vi "GDSLvIcon_GenerateShortClassIconName.vi"(10 "Rows(1)":u8=1, 11 "ClassName":string) -> (3 "ShortClassIconName":string)   [LabVIEW 2012]
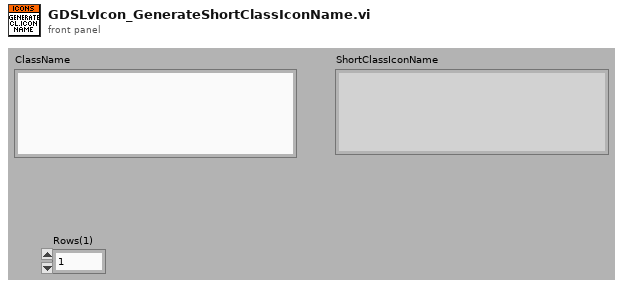
[diagram p1: front panel]
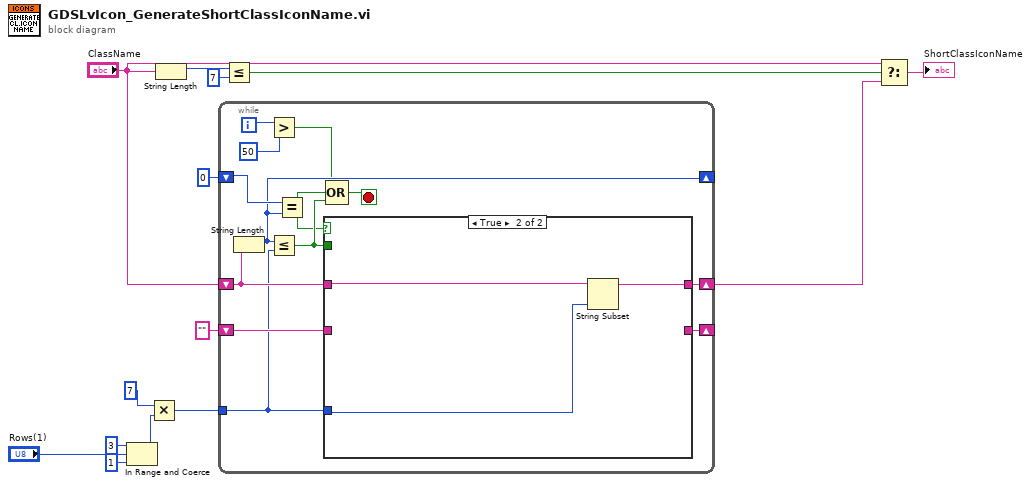
[diagram p0: block diagram]
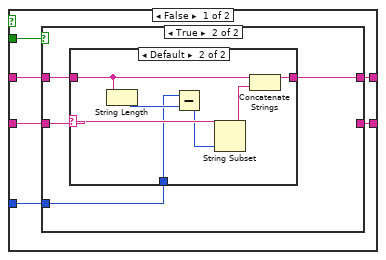
[diagram p2: hidden frame]
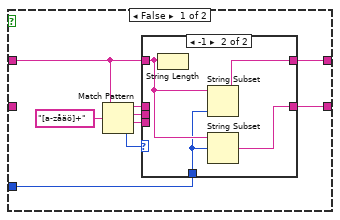
[diagram p3: hidden frame]
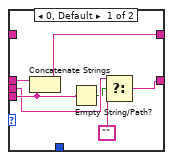
[diagram p4: hidden frame]
diagram:
  n1 = In Range and Coerce(upper limit=u8 3, x="Rows(1)", lower limit=u8 1) -> (coerced(x)=w3:u8)  [unwired: 1 out]
  n2 = Multiply(x=7 ("y"), y=w3) -> (x*y=w1:i32)
  n3 = String Length(string="ClassName") -> (length=w14:i32)
  n4 = while {
    shift-right: [w26] -> w10
    shift-left: "ClassName" -> [w27]
    shift-right: [w24] -> _
    shift-left: 0 -> [w25]
    shift-right: [w20] -> _
    shift-left: "" ("ClassName") -> [w19]
    tunnel: w1 -> [w15]
    i -> [w18]
    stop <- w21 stop-if-true
    n5 = String Length(string=w27) -> (length=w24:i32)
    n6 = Greater?(x=w18, y=50) -> (0:w16:bool)
    n7 = Less Or Equal?(x=w24, y=w15) -> (x <= y?=w23:bool)
    n8 = Equal?(x=w25, y=w24) -> (x = y?=w22:bool)
    n9 = case shown="True" w22 {
      tunnel: w23 -> [w33 _]
      tunnel: w27 -> [w32 w68]
      tunnel: [w31 w67] -> w26
      tunnel: [w30 _] -> w20
      tunnel: w19 -> [w29 _]
      tunnel: w15 -> [w28 w66]
      frame False {
        n10 = case shown="True" w33 {
          tunnel: w32 -> [w37 w56]
          tunnel: [w38 w55] -> w31
          tunnel: [w36 _] -> w30
          tunnel: w29 -> [_ w57]
          tunnel: w28 -> [w34 w54]
          frame False {
            n11 = Match Pattern(string=w37, regular expression="[a-zåäö]+") -> (before substring=w41:string, match substring=w35:string, after substring=w40:string, offset past match=w39:i32)  [unwired: 1 in]
            n12 = case shown="-1" w39 {
              tunnel: w41 -> [w49 _]
              tunnel: w40 -> [w47 _]
              tunnel: [w48 w53] -> w38
              tunnel: w37 -> [_ w52]
              tunnel: [w45 w51] -> w36
              tunnel: w35 -> [w46 _]
              tunnel: w34 -> [_ w50]
              frame 0, Default {
                n13 = Concatenate Strings(w49, w47) -> (w48:string)
                n14 = Empty String/Path?(string/path=w47) -> (empty?=w43:bool)
                n15 = Select(t=w46, s=w43, f="") -> (s? t:f=w45:string)
              }
              frame -1 {
                n16 = String Length(string=w52) -> ()  [unwired: 1 out]
                n17 = String Subset(string=w52, length (rest)=w50) -> (substring=w53:string)  [unwired: 1 in]
                n18 = String Subset(string=w52, offset (0)=w50) -> (substring=w51:string)  [unwired: 1 in]
              }
            }
          }
          frame True {
            n19 = case shown="Default" w57 {
              selector: w57 -> [_ w63]
              tunnel: w56 -> [w58 w65]
              tunnel: [w58 w60] -> w55
              tunnel: w54 -> [_ w59]
              frame "" {
              }
              frame Default {
                n20 = String Length(string=w65) -> (length=w64:i32)
                n21 = Subtract(x=w59, y=w64) -> (x-y=w62:i32)
                n22 = String Subset(string=w63, length (rest)=w62) -> (substring=w61:string)  [unwired: 1 in]
                n23 = Concatenate Strings(w65, w61) -> (w60:string)
              }
            }
          }
        }
      }
      frame True {
        n24 = String Subset(string=w68, length (rest)=w66) -> (substring=w67:string)  [unwired: 1 in]
      }
    }
    n25 = Compound Arithmetic op=OR(w16, w22, w23) -> (w21:bool)
  }
  n26 = Less Or Equal?(x=w14, y=7) -> (x <= y?=w12:bool)
  n27 = Select(t="ClassName", s=w12, f=w10) -> (s? t:f=→"ShortClassIconName":string)
